vi "createConnection.vi"(8 "error in (no error)":errorcluster, 11 "ModernOvenController in":refnum<class "ModernOvenController.lvclass">) -> (0 "error out":errorcluster, 2 "IDeviceConnection":refnum<class "IDeviceConnection.lvclass">, 3 "ModernOvenController out":refnum<class "ModernOvenController.lvclass">)   [LabVIEW 2023, in "ModernOvenController.lvclass"]
doc: "Factory method implementation:\nReturn a new TCPConnection object."
uses:
  ModernOvenController.lvclass
  IDeviceConnection/IDeviceConnection.lvclass
  TCPConnection/TCPConnection.lvclass
  ModernOvenController.lvclass/ModernOvenController.ctl
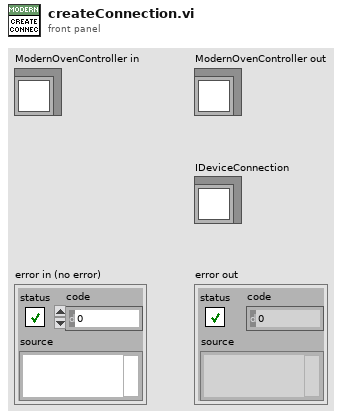
[diagram p1: front panel]
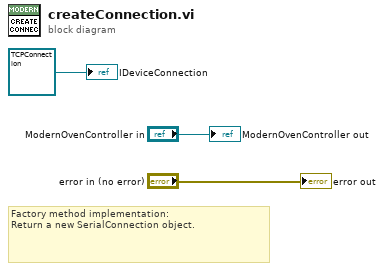
[diagram p0: block diagram]
diagram:
  # "Factory method implementation:\nReturn a new SerialConnection object."
  "error out" <- "error in (no error)"
  "ModernOvenController out" <- "ModernOvenController in"
  "IDeviceConnection" <- refnum<class "TCPConnection.lvclass"> refnum ("TCPConnection.lvclass")
